vi "RT_Controller_Main.vi"() -> ()   [LabVIEW 2020]
uses:
  Components_global/DynamicSignalAnalyzer/TypeDefs/DSA_TF_Enum.ctl
  <vilib>/NI/STM/SubVIs/MetaDataElement.ctl
  <vilib>/NI/STM/TCP/TCP Write Options.ctl
  TypeDefs/STMLoopState_enum.ctl
  <vilib>/Platform/TimedLoop/XDataNode/timing_clust.ctl
  <vilib>/Platform/TimedLoop/XDataNode/nitl_modes.ctl
  <vilib>/Platform/TimedLoop/XDataNode/wakeup.ctl
  Components_global/PlannedMotionSequence/TypeDefs/PlannedMotionSequence.ctl
  Components_global/PlannedMotionSequence/TypeDefs/PlannedMotionSequence_Step.ctl
  Components_global/PlannedMotionSequence/TypeDefs/StepParams.ctl
  Components_global/PlannedMotionSequence/TypeDefs/CtrlEff Params.ctl
  Components_global/PlannedMotionSequence/TypeDefs/PosCtrl Params.ctl
  Components_global/PlannedMotionSequence/TypeDefs/HoldStateParams.ctl
  PC/Controller/TypeDefs/ControllerGains_UI.ctl
  PC/Controller/TypeDefs/ControllerGains_IndAxis.ctl
  Components_global/DynamicSignalAnalyzer/TypeDefs/DSAconfigCluster.ctl
  Components_global/DynamicSignalAnalyzer/TypeDefs/ExcitationSpecs.ctl
  Components_global/DynamicSignalAnalyzer/TypeDefs/CycleSpecs.ctl
  Components_global/DynamicSignalAnalyzer/TypeDefs/DSA_TF_params.ctl
  FPGA/Components/FPGA TypeDefs/SelectDirection_Enum.ctl
  <vilib>/NI/STM/TCP/TCP Read Options.ctl
  TypeDefs/FuncGenParams.ctl
  TypeDefs/SetRefLocEnum.ctl
  FPGA/Components/FPGA TypeDefs/SelectExcitation_Enum.ctl
  Components_global/Queues/InterProcessQueueCtl.ctl
  PC/Controller/TypeDefs/PosZeroOffsets.ctl
  <vilib>/Utility/error.llb/DialogType.ctl
  <vilib>/NI/STM/TCP/Write Meta Data (TCP Ref).vi
  <vilib>/NI/STM/TCP/Get Connection Reference (TCP).vi
  <vilib>/Analysis/2dsp.llb/Unwrap Phase.vi
  <vilib>/NI/STM/TCP/Write Meta Data (TCP Clst).vi
  <vilib>/FPGAPlugInAG/cRIO-9049/niLvFpga_Open_cRIO-9049.vi
  <vilib>/rvi/interface/common/dynamic/niFpgaDynamicAddResources.vi
  <vilib>/Utility/error.llb/Error Cluster From Error Code.vi
  <vilib>/rvi/errors/niLvFpgaAdjustHostInterfaceError.vi
  <vilib>/NI/STM/TCP/Write Message (TCP).vi
  Components_global/DynamicSignalAnalyzer/Private/Cycle_Calculator.vi
  Components_global/DynamicSignalAnalyzer/Private/Take_Data.vi
  Components_global/DynamicSignalAnalyzer/Private/System_Identify.vi
  Components_global/DynamicSignalAnalyzer/Private/Excitation_Gen.vi
  <vilib>/NI/STM/TCP/Read Message (TCP).vi
  <vilib>/FPGAPlugInAG/Dynamic/niLvFpga_Close_Dynamic.vi
  <vilib>/rvi/interface/nirviOpenFPGA/nirviOpenFPGA.xnode
  FPGA Bitfiles/levitationcode_FPGATarget_FPGAmainCtrlv3_XF-7iMJ+Fro.lvbitx
  <vilib>/Platform/TimedLoop/XDataNode/XDataNode.xnode
  <vilib>/rvi/interface/nirviReadWriteControl/nirviReadWriteControl.xnode
  <vilib>/rvi/interface/nirviCloseFPGA/nirviCloseFPGA.xnode
  <vilib>/NI/STM/NI STM.lvlib
  NiFpgaLv.dll
  Components_global/Timing/Timing.lvlib
  <vilib>/Platform/TimedLoop/XDataNode/XDNodeRunTimeDep.lvlib
  Components_global/Queues/Queues.lvlib
  Components_global/DynamicSignalAnalyzer/DynamicSignalAnalyzer.lvlib
  Components/FPGA control IO/FPGAcontrolIO.lvlib
  Components_global/PlannedMotionSequence/PlannedMotionSequence.lvlib
  <vilib>/rvi/interface/Simulation/niFpgaSimulationCallBeginRW.vi
panel:
  out "PlaMoS Iter. Dur. [us]":i64
  out "PlaMoSloop\nFinishedLate Counter":dbl
  out "DSA TF meas":T1
  out "Ts [s]":dbl caption="FPGA Ctrl Loop \nTime (Ts) [s]"
  out "DSAloop\nFinishedLate Counter":dbl
  out "DSAloop Iter. Dur. [us]":i64
  out "ReadLoop FinishedLate Counter":dbl
  out "ReadLoop Iteration \nDuration (us)":i64
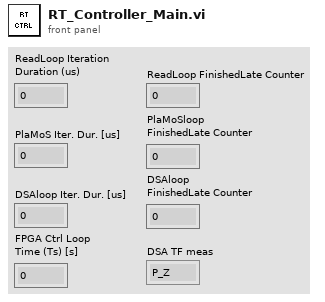
[diagram p1: front panel]
types:
  T1 = typedef "DynamicSignalAnalyzer.lvlib/DSA_TF_Enum.ctl" = enum16{"P_Z", "P_ThX", "P_ThY", "P_Bow", "P_B-d", "C_Z", "C_ThX", "C_ThY", "C_Bow", "C_B-d", "RR_Z", "RR_ThX", "RR_ThY", "RR_Bow", "RR_B-d", "*_custom"}
  T2 = typedef "STMLoopState_enum.ctl" = enum16{"Initialize", "Warm-up", "Run", "ShutDown"}
  T3 = typedef "NI STM.lvlib/TCP Write Options.ctl" = cluster{"ignore timeout error":bool, "timeout ms (1000)":i32}
  T4 = typedef "NI STM.lvlib/MetaDataElement.ctl" = string
  T5 = typedef "NI STM.lvlib/TCP Connection Info.ctl" = cluster{"connection ID":refnum<k5>, "meta data":T4[]}
  T6 = typedef "Queues.lvlib/Queue Refs.ctl" = cluster{"InterProcessQueue":refnum<queue>}
  T7 = typedef "XDNodeRunTimeDep.lvlib/timing_clust.ctl" = cluster{"Expected End [f-1]":u64, "Actual End [f-1]":u64, "Finished Late? [f-1]":bool, "Expected End [i-1]":u64, "Actual End [i-1]":u64, "Finished Late? [i-1]":bool, "Expected Start [i]":u64, "Actual Start [i]":u64, "Expected Start [f]":u64, "Actual Start [f]":u64, "Source Name":string, "Structure Name":string, "Period":i64, "Deadline":i64, "Offset":i64, "Start":i64, "Priority":i32, "Timeout":i32, "Mode":T8, "Wakeup Reason":T9, "Error":errorcluster, "Source Type":string, "Secondary Source Type":string, "Global End Time":u64, "Global Start Time":u64, "Frame Duration":u64, "Iteration Duration":u64, "Assigned CPU":i32, "I/O Scan Engine Mode":u32}
  T8 = typedef "XDNodeRunTimeDep.lvlib/nitl_modes.ctl" = enum32{"No Change", "Process missed periods, maintain original phase", "Discard missed periods, maintain original phase", "Process missed periods, ignore original phase", "Discard missed periods, ignore original phase"}
  T9 = typedef "XDNodeRunTimeDep.lvlib/wakeup.ctl" = enum32{"Normal", "Aborted", "Asynchronous wakeup", "Timing source error", "Timed loop error", "Timeout"}
  T10 = typedef "PlannedMotionSequence.lvlib/PlannedMotionSequence.ctl" = T11[]
  T11 = typedef "PlannedMotionSequence.lvlib/PlannedMotionSequence_Step.ctl" = cluster{"_Comment":string, "StepParams":T12, "Controller Gains":T16}
  T12 = typedef "PlannedMotionSequence.lvlib/StepParams.ctl" = cluster{"Ctrl State":enum16{"PosCtrl", "CtrlEff", "HoldState"}, "CtrlEff Params":T13, "PosCtrl Params":T14, "HoldState Params":T15}
  T13 = typedef "PlannedMotionSequence.lvlib/CtrlEff Params.ctl" = cluster{"Time [s]":dbl, "U_z":dbl}
  T14 = typedef "PlannedMotionSequence.lvlib/PosCtrl Params.ctl" = cluster{"Velocity [um/s]":dbl, "Starting Z-position [um]":dbl, "Ending Z-position [um]":dbl, "Bow Reference [um]":dbl}
  T15 = typedef "PlannedMotionSequence.lvlib/HoldStateParams.ctl" = cluster{"Time [s]":dbl}
  T16 = typedef "ControllerGains_UI.ctl" = cluster{"Z-direction":T17, "ThX-direction":T17, "ThY-direction":T17, "Bow-direction":T17, "Tor-direction":T17}
  T17 = typedef "ControllerGains_IndAxis.ctl" = cluster{"Kp":dbl, "Ki":dbl, "fLPF":dbl}
  T18 = cluster{"Period":i64, "State Index":i32, "index":i32}
  T19 = typedef "DynamicSignalAnalyzer.lvlib/DSAconfigCluster.ctl" = cluster{"DSA excitation specs":T20, "Cycle Specs":T21, "Meas. TF params":T22}
  T20 = typedef "DynamicSignalAnalyzer.lvlib/ExcitationSpecs.ctl" = cluster{"Initial Freq. [Hz]":dbl, "Final Freq. [Hz]":dbl, "# pts. in interval":i16, "Samping Time [us]":dbl, "Amplitude":dbl, "Offset [V]":dbl, "Freq Units (F: rad/s, T: Hz)":bool}
  T21 = typedef "DynamicSignalAnalyzer.lvlib/CycleSpecs.ctl" = cluster{"Cycles To \nSettle (M)":i16, "Cycles To \nCalculate (N)":i16}
  T22 = typedef "DynamicSignalAnalyzer.lvlib/DSA_TF_params.ctl" = cluster{"Direction":T23, "Tras. Func.":enum16{"P", "RR", "C", "*_custom"}}
  T23 = typedef "SelectDirection_Enum.ctl" = enum8{"Z", "ThX", "ThY", "Bow", "Tor"}
  T24 = typedef "NI STM.lvlib/TCP Read Options.ctl" = cluster{"ignore timeout error":bool, "timeout ms (1000)":i32}
  T25 = typedef "FuncGenParams.ctl" = cluster{"Reference Location":T26, "Direction":T23, "Excitation mode":T27, "Amplitude":dbl, "Frequency (periods/tick)":dbl, "PosRef_Offset":dbl[]}
  T26 = typedef "SetRefLocEnum.ctl" = enum16{"Pos Ref", "Ctrl Eff", "Elec Volt Dist"}
  T27 = typedef "SelectExcitation_Enum.ctl" = enum8{"DC", "Sine", "Square", "WhiteNoise"}
  T28 = typedef "Queues.lvlib/InterProcessQueueCtl.ctl" = cluster{"Command":string, "Data":variant}
  T29 = typedef "PosZeroOffsets.ctl" = cluster{"V_SE":dbl, "V_NE":dbl, "V_NW":dbl, "V_SW":dbl, "V_CI":dbl}
  T30 = cluster{"[0]":dbl, "[1]":dbl, "[2]":dbl, "[3]":dbl, "[4]":dbl}
  T31 = cluster{"[0]":dbl, "[1]":dbl, "[2]":dbl, "[3]":dbl, "[4]":dbl, "[5]":dbl}
  T32 = typedef "DialogType.ctl" = u16
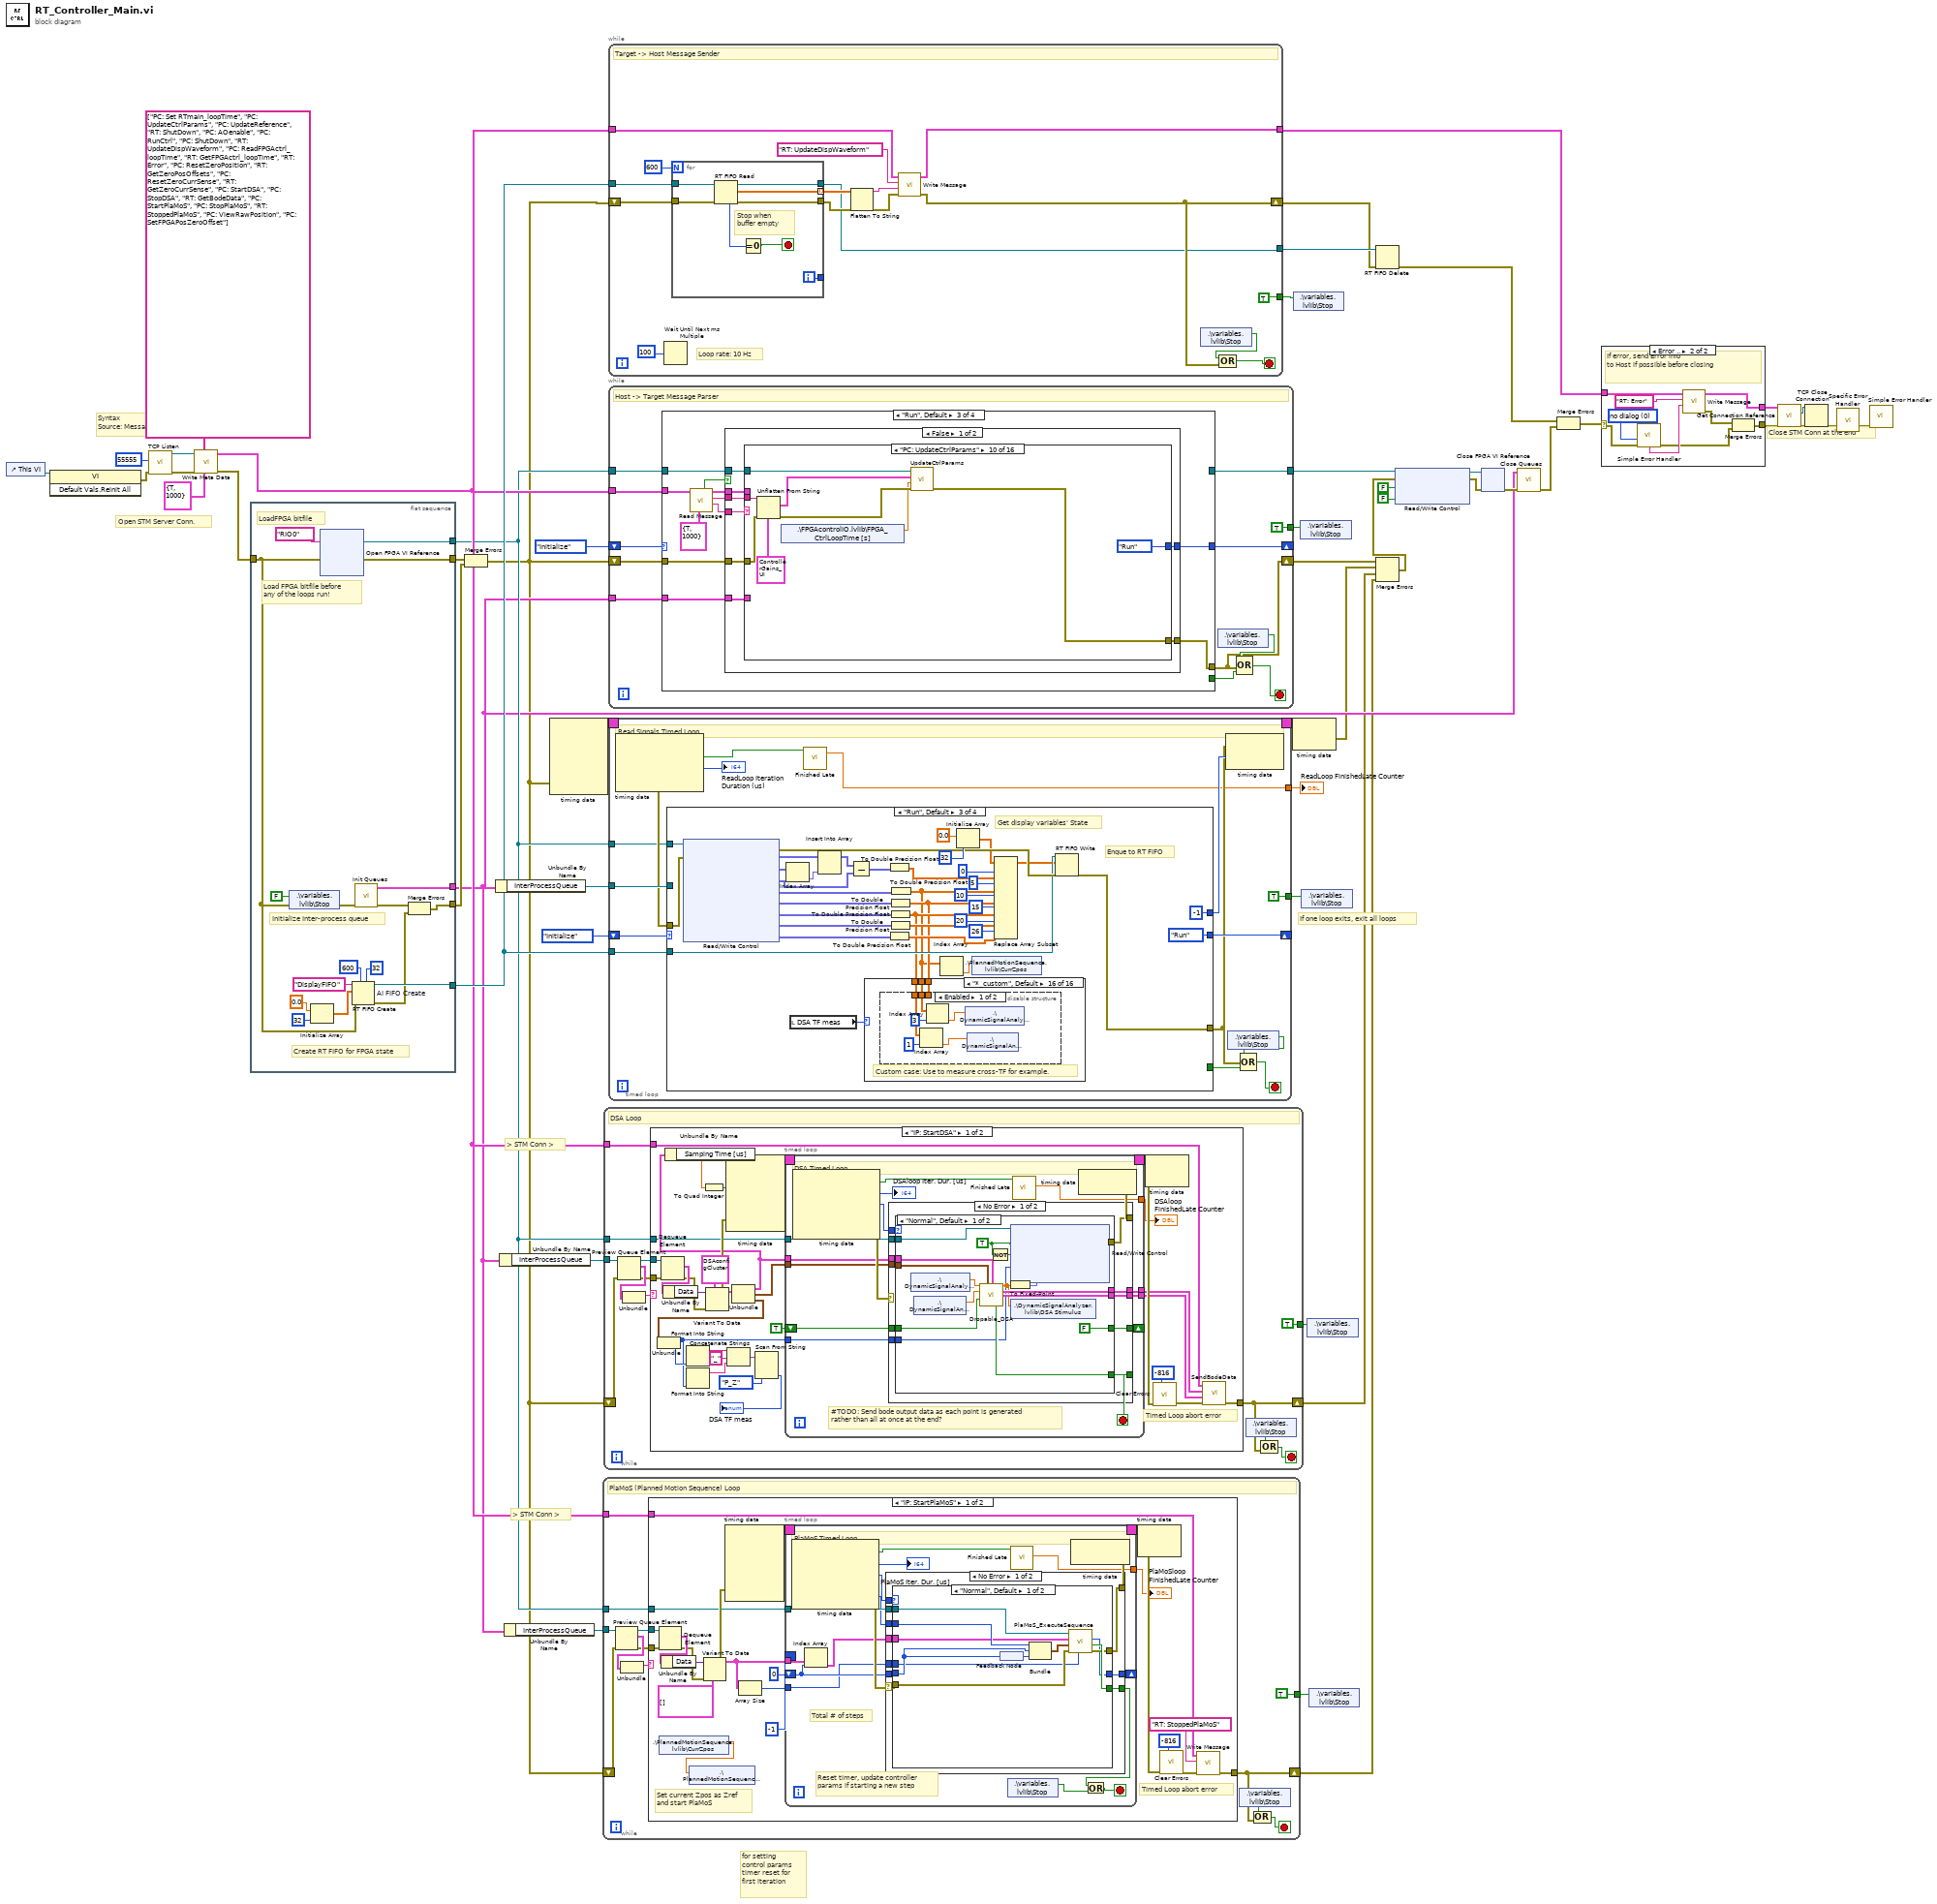
[diagram p0: block diagram]
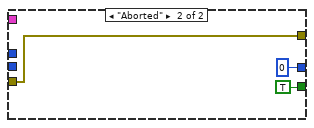
[diagram p2: hidden frame]
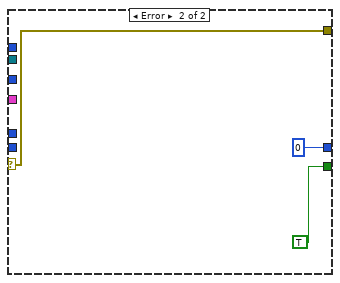
[diagram p3: hidden frame]
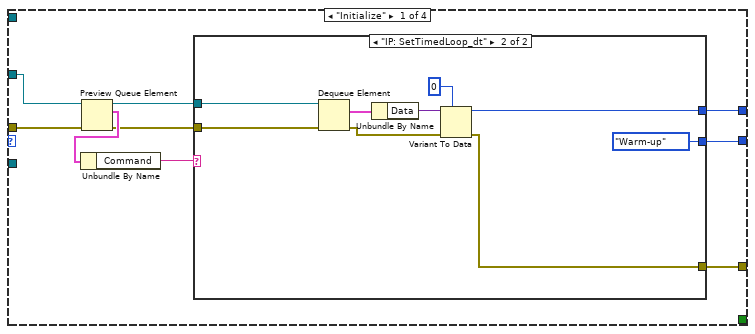
[diagram p5: hidden frame]
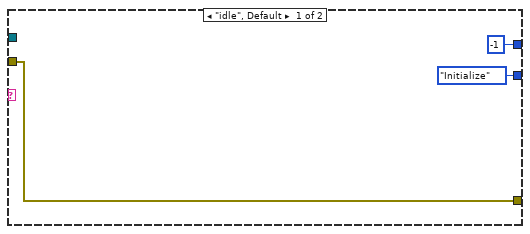
[diagram p6: hidden frame]
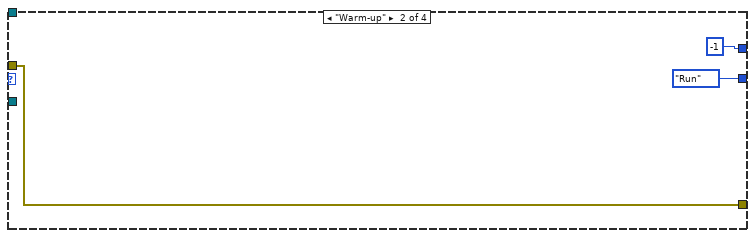
[diagram p7: hidden frame]
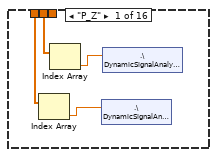
[diagram p8: hidden frame]
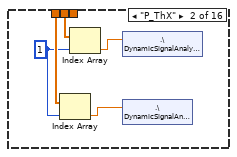
[diagram p9: hidden frame]
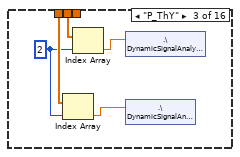
[diagram p10: hidden frame]
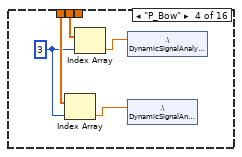
[diagram p11: hidden frame]
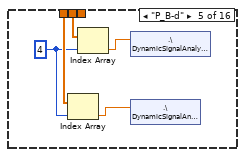
[diagram p12: hidden frame]
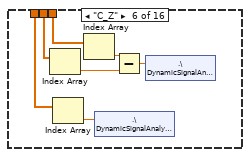
[diagram p13: hidden frame]
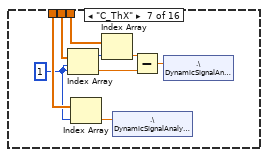
[diagram p14: hidden frame]
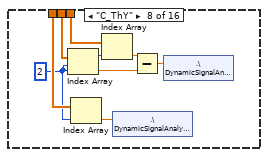
[diagram p15: hidden frame]
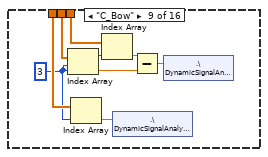
[diagram p16: hidden frame]
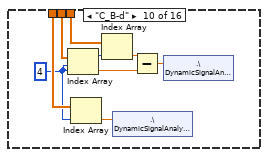
[diagram p17: hidden frame]
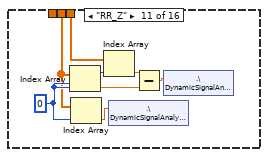
[diagram p18: hidden frame]
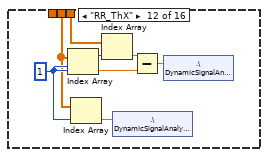
[diagram p19: hidden frame]
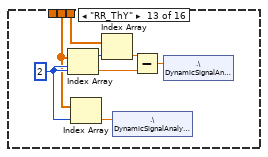
[diagram p20: hidden frame]
diagram:
  # "for setting control params\ntimer reset for\nfirst iteration"
  # "> STM Conn >"
  # "> STM Conn >"
  # "Close STM Conn at the end"
  # "Syntax\nSource: Message"
  # "Open STM Server Conn."
  # "If one loop exits, exit all loops"
  n1 = control-ref of="This VI"() -> (w13:refnum<vi>)
  n2 = invoke on="Invoke Node" class="VI" method="Default Vals.Reinit All"(reference=w13) -> (error out=w12:errorcluster)  [unwired: 2 in, 2 out]
  n3 = call <vilib>:"TCP Listen.vi"("error in (no error)"=w12, "port"=u16 55555) -> ("error out"=w50:errorcluster, "connection ID"=w49:refnum<k5>)  [unwired: 5 in, 3 out]
  n4 = call-poly <vilib>:"Write Meta Data.vi"("options"=T3 {"ignore timeout error"=TRUE, "timeout ms (1000)"=1000}, "meta data"=T4[] ["PC: Set RTmain_loopTime", "PC: UpdateCtrlParams", "PC: UpdateReference", "RT: ShutDown", "PC: AOenable", "PC: RunCtrl", "PC: ShutDown", "RT: UpdateDispWaveform", "PC: ReadFPGActrl_loopTime", "RT: GetFPGActrl_loopTime", "RT: Error", "PC: ResetZeroPosition", "RT: GetZeroPosOffsets", "PC: ResetZeroCurrSense", "RT: GetZeroCurrSense", "PC: StartDSA", "PC: StopDSA", "RT: GetBodeData", "PC: StartPlaMoS", "PC: StopPlaMoS", "RT: StoppedPlaMoS", "PC: ViewRawPosition", "PC: SetFPGAPosZeroOffset"], "error in"=w50, "connection ID"=w49) -> ("error out"=w45:errorcluster, "connection info out"=w9:T5)  [unwired: 1 in, 5 out]
  n5 = flat-sequence {
    tunnel: w45 -> [w53]
    tunnel: [w52] -> w8
    tunnel: [w68] -> w41
    tunnel: [w66] -> w6
    tunnel: [w56] -> w40
    tunnel: [w59] -> w36
    frame #0 {
      # "Create RT FIFO for FPGA state"
      # "LoadFPGA bitfile"
      # "Initialize Inter-process queue"
      # "Load FPGA bitfile before \nany of the loops run!"
      n6 = shared-variable ".\\variables.lvlib\\Stop"(FALSE ("Stop"), error in=w53) -> (error out=w58:errorcluster)
      n7 = Initialize Array(0.0 ("element"), 32 ("dimension size")) -> (w61:dbl[])
      n8 = xnode "Open FPGA VI Reference"("error in"=w53, "resource name"=tag "RIO0") -> ("FPGA VI Reference Out"=w52:refnum<k20>, "error out"=w68:errorcluster)
      n9 = RT FIFO Create "AI FIFO Create"(0:"DisplayFIFO" ("name (unnamed)"), 1:w61, 3:w53, 4:u32 600 ("size (10)"), 6:u32 32 ("elements in array (1)")) -> (8:w59:refnum<k33>, 11:w54:errorcluster)  [unwired: 3 in, 1 out]
      n10 = call "Init Queues.vi"("error in (no error)"=w58) -> ("error out"=w55:errorcluster, "Queue Refs"=w66:T6)  [unwired: 9 in]
      n11 = Merge Errors(w55, w54) -> (w56:errorcluster)
    }
  }
  n12 = Merge Errors(w41, w40) -> (w1:errorcluster)
  n13 = Unbundle By Name(w6) -> ("InterProcessQueue"=w39:refnum<queue>)
  n14 = Unbundle By Name(w6) -> ("InterProcessQueue"=w16:refnum<queue>)
  n15 = Unbundle By Name(w6) -> ("InterProcessQueue"=w11:refnum<queue>)
  n16 = node-c288(w1) -> (w44:T7)  [unwired: 4 in]
  n17 = while {
    tunnel: w11 -> [w80]
    tunnel: [TRUE ("Stop")] -> w10
    shift-right: [w71] -> w2
    shift-left: w1 -> [w73]
    tunnel: w9 -> [w70]
    tunnel: w8 -> [w69]
    stop <- w79 stop-if-true
    # "PlaMoS (Planned Motion Sequence) Loop"
    n18 = Preview Queue Element(queue=w80, error in (no error)=w73) -> (queue out=w74:refnum<queue>, element=w76:cluster{"Command":string, "Data":variant}, error out=w72:errorcluster)  [unwired: 1 in, 1 out]
    n19 = Unbundle(w76) -> ("Command"=w75:string)  [unwired: 1 out]
    n20 = case shown="\"IP: StartPlaMoS\"" w75 {
      tunnel: w74 -> [w100 _]
      tunnel: w72 -> [w99 w160]
      tunnel: [w91 w160] -> w71
      tunnel: w70 -> [w90 _]
      tunnel: w69 -> [w89 _]
      frame "IP: StartPlaMoS" {
        # "Set current Zpos as Zref \nand start PlaMoS"
        # "Timed Loop abort error"
        n21 = Dequeue Element(queue=w100, error in (no error)=w99) -> (element=w98:cluster{"Command":string, "Data":variant}, error out=w96:errorcluster)  [unwired: 1 in, 2 out]
        n22 = shared-variable ".\\PlannedMotionSequence.lvlib\\CurrZpos"() -> (w81:dbl)  [unwired: 1 in, 1 out]
        n23 = Unbundle By Name(w98) -> ("Data"=w97:variant)
        n24 = shared-variable ".\\PlannedMotionSequence.lvlib\\CurrZref"(w81) -> ()  [unwired: 1 in, 1 out]
        n25 = Variant To Data(error in=w96, type=T10 [] ("Planned Motion Sequence Steps"), Variant=w97) -> (data=w83:T10, error out=w95:errorcluster)
        n26 = node-c288(w95) -> (w102:T7)  [unwired: 4 in]
        n27 = Array Size(array=w83) -> (size(s)=w84:i32)
        n28 = timed-loop {
          timing: w102 -> [_]
          timing-out: [_] -> w101
          tunnel: w89 -> [w115]
          tunnel: [w113] -> w88
          tunnel: w83 -> [w108]
          shift-right: [w111] -> _
          shift-left: 0 ("State Index") -> [w109]
          tunnel: w84 -> [w107]
          border: -1 ("index") -> [_]
          stop <- w106 stop-if-true
          # "Reset timer, update controller params if starting a new step"
          # "Total # of steps"
          # "PlaMoS Timed Loop"
          n29 = node-c288() -> (w114:bool, →"PlaMoS Iter. Dur. [us]":i64, w118:T9, w117:errorcluster, w110:i64)  [unwired: 1 in]
          n30 = Index Array(array=w108, index=w109) -> (element=w103:T11)
          n31 = case shown="No Error" w117 {
            selector: w117 -> [w125 w145]
            tunnel: w118 -> [w128 _]
            tunnel: [w127 TRUE] -> w105
            tunnel: [w121 w145] -> w116
            tunnel: w115 -> [w126 _]
            tunnel: w109 -> [w124 _]
            tunnel: [w123 0 ("Next State Index")] -> w111
            tunnel: w110 -> [w122 _]
            tunnel: w107 -> [w120 _]
            tunnel: w103 -> [w119 _]
            frame No Error {
              n32 = case shown="\"Normal\", Default" w128 {
                tunnel: [w138 TRUE] -> w127
                tunnel: w126 -> [w134 _]
                tunnel: w125 -> [w139 w140]
                tunnel: w124 -> [w135 _]
                tunnel: [w131 0 ("Next State Index")] -> w123
                tunnel: w122 -> [w137 _]
                tunnel: [w133 w140] -> w121
                tunnel: w120 -> [w132 _]
                tunnel: w119 -> [w129 _]
                frame "Normal", Default {
                  n33 = feedback-in #1(w135) -> ()
                  n34 = feedback #1() -> (w130:i32)
                  n35 = Bundle("Period"=w137, "State Index"=w135, "index"=w130) -> (w136:T18)  [unwired: 1 in]
                  n36 = call "PlaMoS_ExecuteSequence.vi"("Total # of seq steps"=w132, "error in (no error)"=w139, "Curr Iter Params"=w136, "PlannedMotionSequence Step"=w129, "FPGA VI Reference In"=w134) -> ("error out"=w133:errorcluster, "PlaMoS completed?"=w138:bool, "Next State Index"=w131:i32)  [unwired: 3 in, 1 out]
                }
                frame "Aborted" {
                }
              }
            }
            frame Error {
            }
          }
          n37 = shared-variable ".\\variables.lvlib\\Stop"() -> (w104:bool)  [unwired: 1 in, 1 out]
          n38 = call "Finished Late.vi"("Finished \nLate?"=w114) -> ("# Finished\nLate counter"=w113:dbl)  [unwired: 8 in, 2 out]
          n39 = node-c288(w116) -> ()  [unwired: 1 out]
          n40 = Or(x=w105, y=w104) -> (x .or. y?=w106:bool)
        }
        "PlaMoSloop\nFinishedLate Counter" <- w88
        n41 = node-c288(w101) -> (w93:errorcluster)
        n42 = call <vilib>:"Clear Errors.vi"("error in (no error)"=w93, "specific error code to clear (0: all)"=-816) -> ("error out"=w92:errorcluster)  [unwired: 4 in, 1 out]
        n43 = call-poly <vilib>:"Write Message.vi"("error in"=w92, "name"="RT: StoppedPlaMoS", "connection info in"=w90) -> ("error out"=w91:errorcluster)  [unwired: 7 in, 1 out]
      }
      frame "idle", Default {
      }
    }
    n44 = shared-variable ".\\variables.lvlib\\Stop"() -> (w78:bool)  [unwired: 1 in, 1 out]
    n45 = Compound Arithmetic op=OR(w78, w71) -> (w79:bool)
  }
  n46 = while {
    tunnel: w16 -> [w172]
    tunnel: [TRUE ("Stop")] -> w15
    shift-right: [w163] -> w3
    shift-left: w1 -> [w165]
    tunnel: w9 -> [w162]
    tunnel: w8 -> [w161]
    stop <- w171 stop-if-true
    # "DSA Loop"
    n47 = Preview Queue Element(queue=w172, error in (no error)=w165) -> (queue out=w166:refnum<queue>, element=w168:cluster{"Command":string, "Data":variant}, error out=w164:errorcluster)  [unwired: 1 in, 1 out]
    n48 = Unbundle(w168) -> ("Command"=w167:string)  [unwired: 1 out]
    n49 = case shown="\"IP: StartDSA\"" w167 {
      tunnel: w166 -> [w203 _]
      tunnel: w164 -> [w202 w265]
      tunnel: [w187 w265] -> w163
      tunnel: w162 -> [w184 _]
      tunnel: w161 -> [w183 _]
      frame "IP: StartDSA" {
        # "Timed Loop abort error"
        n50 = Dequeue Element(queue=w203, error in (no error)=w202) -> (element=w201:cluster{"Command":string, "Data":variant}, error out=w198:errorcluster)  [unwired: 1 in, 2 out]
        n51 = Unbundle By Name(w201) -> ("Data"=w200:variant)
        n52 = Variant To Data(error in=w198, type=T19 {"DSA excitation specs"={"Initial Freq. [Hz]"=1.0, "Final Freq. [Hz]"=100.0, "# pts. in interval"=20, "Samping Time [us]"=0.0, "Amplitude"=0.0003, "Offset [V]"=0.0, "Freq Units (F: rad/s, T: Hz)"=TRUE}, "Cycle Specs"={"Cycles To \nSettle (M)"=1, "Cycles To \nCalculate (N)"=2}, "Meas. TF params"={"Direction"=enum."Z", "Tras. Func."=enum."P"}} ("DSA Config Cluster"), Variant=w200) -> (data=w195:T19, error out=w197:errorcluster)
        n53 = Unbundle(w195) -> ("DSA excitation specs"=w192:T20, "Cycle Specs"=w191:T21, "Meas. TF params"=w181:T22)
        n54 = Unbundle(w181) -> ("Direction"=w173:T23, "Tras. Func."=w180:enum16{"P", "RR", "C", "*_custom"})
        n55 = Unbundle By Name(w192) -> ("Samping Time [us]"=w189:dbl)
        n56 = Format Into String(w180) -> (resulting string=w179:string)  [unwired: 3 in, 1 out]
        n57 = Format Into String(w173) -> (resulting string=w177:string)  [unwired: 3 in, 1 out]
        n58 = To Quad Integer(1:w189) -> (0:w190:i64)
        n59 = node-c288(w190, w197) -> (w205:T7)  [unwired: 3 in]
        n60 = Concatenate Strings(w179, "_" ("string"), w177) -> (w176:string)
        n61 = Scan From String(input string=w176, default 1=DSA_TF_Enum."P_Z") -> (output 1=→"DSA TF meas":T1)  [unwired: 3 in, 3 out]
        n62 = timed-loop {
          timing: w205 -> [_]
          timing-out: [_] -> w204
          shift-right: [w215] -> _
          shift-left: TRUE ("START") -> [w216]
          tunnel: w192 -> [w214]
          tunnel: w191 -> [w213]
          tunnel: [w212] -> w186
          tunnel: [w211] -> w185
          tunnel: w183 -> [w209]
          tunnel: [w207] -> w182
          tunnel: w173 -> [w206]
          stop <- w219 stop-if-true
          # "#TODO: Send bode output data as each point is generated \nrather than all at once at the end?"
          # "DSA Timed Loop"
          n63 = node-c288() -> (w208:bool, →"DSAloop Iter. Dur. [us]":i64, w220:T9, w218:errorcluster)  [unwired: 1 in, 1 out]
          n64 = case shown="No Error" w218 {
            selector: w218 -> [_ w250]
            tunnel: w220 -> [w231 _]
            tunnel: [w230 TRUE] -> w219
            tunnel: [w222 w250] -> w217
            tunnel: w216 -> [w229 _]
            tunnel: [w228 _] -> w215
            tunnel: w214 -> [w227 _]
            tunnel: w213 -> [w226 _]
            tunnel: [w225 _] -> w212
            tunnel: [w224 _] -> w211
            tunnel: w209 -> [w223 _]
            tunnel: w206 -> [w221 _]
            frame No Error {
              n65 = case shown="\"Normal\", Default" w231 {
                tunnel: [w244 TRUE] -> w230
                tunnel: w229 -> [w243 _]
                tunnel: [FALSE ("START") _] -> w228
                tunnel: w227 -> [w242 _]
                tunnel: w226 -> [w241 _]
                tunnel: [w240 _] -> w225
                tunnel: [w239 _] -> w224
                tunnel: w223 -> [w238 _]
                tunnel: [w237 _] -> w222
                tunnel: w221 -> [w232 _]
                frame "Normal", Default {
                  w234 = TRUE ("Enable  Ctrl Eff dist?")
                  n66 = shared-variable ".\\DynamicSignalAnalyzer.lvlib\\TF Out"() -> (w247:dbl)  [unwired: 1 in, 1 out]
                  n67 = shared-variable ".\\DynamicSignalAnalyzer.lvlib\\TF In"() -> (w246:dbl)  [unwired: 1 in, 1 out]
                  n68 = call "Dropable_DSA.vi"("TF Out (CH B)"=w247, "Cycle Specs"=w241, "Excitation Specs"=w242, "TF In (CH A)"=w246, "START"=w243) -> ("Disturbance"=w236:dbl, "Bode Magnitude"=w240:cluster{dbl[], dbl[]}, "Bode Phase"=w239:cluster{dbl[], dbl[]}, "Stopped"=w244:bool)  [unwired: 5 in, 2 out]
                  n69 = Not(x=w234) -> (.not. x?=w235:bool)
                  n70 = To Fixed-Point(number=w236) -> (fixed-point=w233:fxp<+/-,25,5>)  [unwired: 1 in]
                  n71 = xnode "Read/Write Control"("FPGA VI Reference In"=w238, "Enable  Pos. Ref. Gen?"=w234, "Enable  Ctrl Eff dist?"=w235, "Select Ref. direction"=w232, "PR Amplitude [V]"=w233) -> ("error out"=w237:errorcluster)  [unwired: 1 in, 1 out]
                  n72 = shared-variable ".\\DynamicSignalAnalyzer.lvlib\\DSA Stimulus"(w236) -> ()  [unwired: 1 in, 1 out]
                }
                frame "Aborted" {
                }
              }
            }
            frame Error {
            }
          }
          n73 = call "Finished Late.vi"("Finished \nLate?"=w208) -> ("# Finished\nLate counter"=w207:dbl)  [unwired: 8 in, 2 out]
          n74 = node-c288(w217) -> ()  [unwired: 1 out]
        }
        "DSAloop\nFinishedLate Counter" <- w182
        n75 = node-c288(w204) -> (w193:errorcluster)
        n76 = call <vilib>:"Clear Errors.vi"("error in (no error)"=w193, "specific error code to clear (0: all)"=-816) -> ("error out"=w188:errorcluster)  [unwired: 4 in, 1 out]
        n77 = call "SendBodeData.vi"("error in (no error)"=w188, "Phase Array"=w185, "Magnitude Array"=w186, "connection info in"=w184) -> ("error out"=w187:errorcluster)  [unwired: 6 in, 1 out]
      }
      frame "idle", Default {
      }
    }
    n78 = shared-variable ".\\variables.lvlib\\Stop"() -> (w170:bool)  [unwired: 1 in, 1 out]
    n79 = Compound Arithmetic op=OR(w170, w163) -> (w171:bool)
  }
  n80 = timed-loop {
    timing: w44 -> [_]
    timing-out: [_] -> w43
    shift-right: [w279] -> _
    shift-left: STMLoopState_enum."Initialize" ("RTmainLoopState") -> [w280]
    tunnel: w39 -> [w276]
    tunnel: [TRUE ("Stop")] -> w38
    tunnel: w36 -> [w268]
    tunnel: w8 -> [w267]
    tunnel: [w266] -> w18
    stop <- w273 stop-if-true
    # "Read Signals Timed Loop"
    n81 = node-c288() -> (w274:errorcluster, w278:bool, →"ReadLoop Iteration \nDuration (us)":i64)  [unwired: 1 in, 1 out]
    n82 = case shown="\"Run\", Default" w280 {
      tunnel: [w286 STMLoopState_enum."Run" ("RTmainLoopState") STMLoopState_enum."Run" ("RTmainLoopState") STMLoopState_enum."ShutDown" ("RTmainLoopState")] -> w279
      tunnel: [_ _ _ TRUE] -> w272
      tunnel: w276 -> [w285 _ _ _]
      tunnel: [w284 i64 -1 ("Period") i64 -1 ("Period") i64 1000 ("Period")] -> w275
      tunnel: w274 -> [w283 w302 w337 w456]
      tunnel: [w281 w302 w330 w456] -> w271
      tunnel: w268 -> [_ _ w329 _]
      tunnel: w267 -> [_ _ w338 _]
      frame "Initialize" {
        n83 = Preview Queue Element(queue=w285, error in (no error)=w283) -> (queue out=w289:refnum<queue>, element=w288:cluster{"Command":string, "Data":variant}, error out=w282:errorcluster)  [unwired: 1 in, 1 out]
        n84 = Unbundle By Name(w288) -> ("Command"=w287:string)
        n85 = case shown="\"IP: SetTimedLoop_dt\"" w287 {
          tunnel: w289 -> [_ w300]
          tunnel: [STMLoopState_enum."Initialize" ("RTmainLoopState") STMLoopState_enum."Warm-up" ("RTmainLoopState")] -> w286
          tunnel: [i64 -1 w296] -> w284
          tunnel: w282 -> [w290 w295]
          tunnel: [w290 w293] -> w281
          frame "idle", Default {
          }
          frame "IP: SetTimedLoop_dt" {
            n86 = Dequeue Element(queue=w300, error in (no error)=w295) -> (element=w299:cluster{"Command":string, "Data":variant}, error out=w294:errorcluster)  [unwired: 1 in, 2 out]
            n87 = Unbundle By Name(w299) -> ("Data"=w298:variant)
            n88 = Variant To Data(error in=w294, type=i64 0, Variant=w298) -> (data=w296:i64, error out=w293:errorcluster)
          }
        }
      }
      frame "Warm-up" {
      }
      frame "Run", Default {
        # "Enque to RT FIFO"
        # "Get display variables' State"
        n89 = xnode "Read/Write Control"("FPGA VI Reference In"=w338, "error in"=w337) -> ("error out"=w331:errorcluster, "AI_HS"=w325:fxp<+/-,25,5>[], "AI_LS"=w327:fxp<+/-,25,5>[], "PosMeas_ZeroOffset"=w326:fxp<+/-,25,5>[], "Z,ThX,ThY,B,Bd Meas"=w310:fxp<+/-,25,5>[], "Total PosRef"=w336:fxp<+/-,25,5>[], "Total Ctrl Eff"=w335:fxp<+/-,25,5>[], "AO"=w334:fxp<+/-,20,5>[], "Current Sense"=w328:fxp<+/-,25,5>[])  [unwired: 1 out]
        n90 = Index Array(array=w327) -> (element=w324:fxp<+/-,25,5>)  [unwired: 1 in]
        n91 = local read "DSA TF meas"() -> (w307:T1)
        n92 = Insert Into Array(array=w325, new element=w324) -> (w323:fxp<+/-,25,5>[])  [unwired: 1 in]
        n93 = Subtract(x=w323, y=w326) -> (x-y=w322:fxp<+/-,26,6>[])
        n94 = To Double Precision Float(number=w322) -> (double precision float=w320:dbl[])
        n95 = To Double Precision Float(number=w328) -> (double precision float=w313:dbl[])
        n96 = To Double Precision Float(number=w336) -> (double precision float=w308:dbl[])
        n97 = To Double Precision Float(number=w335) -> (double precision float=w309:dbl[])
        n98 = To Double Precision Float(number=w334) -> (double precision float=w314:dbl[])
        n99 = To Double Precision Float(number=w310) -> (double precision float=w305:dbl[])
        n100 = case shown="\"*_custom\", Default" w307 {
          tunnel: w305 -> [w343 w348 w353 w358 w363 w371 w379 w387 w395 w403 w404 w411 w418 w425 w432 w441]
          tunnel: w309 -> [w341 w346 w351 w356 w361 w365 w373 w381 w389 w397 _ _ _ _ _ w440]
          tunnel: w308 -> [_ _ _ _ _ w367 w375 w383 w391 w399 w407 w414 w421 w428 w435 w439]
          frame "P_Z" {
            n101 = Index Array(array=w341) -> (element=w342:dbl)  [unwired: 1 in]
            n102 = Index Array(array=w343) -> (element=w344:dbl)  [unwired: 1 in]
            n103 = shared-variable ".\\DynamicSignalAnalyzer.lvlib\\TF In"(w342) -> ()  [unwired: 1 in, 1 out]
            n104 = shared-variable ".\\DynamicSignalAnalyzer.lvlib\\TF Out"(w344) -> ()  [unwired: 1 in, 1 out]
          }
          frame "P_ThX" {
            w345 = 1 ("index")
            n105 = Index Array(array=w346, index=w345) -> (element=w347:dbl)
            n106 = Index Array(array=w348, index=w345) -> (element=w349:dbl)
            n107 = shared-variable ".\\DynamicSignalAnalyzer.lvlib\\TF Out"(w349) -> ()  [unwired: 1 in, 1 out]
            n108 = shared-variable ".\\DynamicSignalAnalyzer.lvlib\\TF In"(w347) -> ()  [unwired: 1 in, 1 out]
          }
          frame "P_ThY" {
            w350 = 2 ("index")
            n109 = Index Array(array=w351, index=w350) -> (element=w352:dbl)
            n110 = Index Array(array=w353, index=w350) -> (element=w354:dbl)
            n111 = shared-variable ".\\DynamicSignalAnalyzer.lvlib\\TF Out"(w354) -> ()  [unwired: 1 in, 1 out]
            n112 = shared-variable ".\\DynamicSignalAnalyzer.lvlib\\TF In"(w352) -> ()  [unwired: 1 in, 1 out]
          }
          frame "P_Bow" {
            w355 = 3 ("index")
            n113 = Index Array(array=w356, index=w355) -> (element=w357:dbl)
            n114 = Index Array(array=w358, index=w355) -> (element=w359:dbl)
            n115 = shared-variable ".\\DynamicSignalAnalyzer.lvlib\\TF Out"(w359) -> ()  [unwired: 1 in, 1 out]
            n116 = shared-variable ".\\DynamicSignalAnalyzer.lvlib\\TF In"(w357) -> ()  [unwired: 1 in, 1 out]
          }
          frame "P_B-d" {
            w360 = 4 ("index")
            n117 = Index Array(array=w361, index=w360) -> (element=w362:dbl)
            n118 = Index Array(array=w363, index=w360) -> (element=w364:dbl)
            n119 = shared-variable ".\\DynamicSignalAnalyzer.lvlib\\TF Out"(w364) -> ()  [unwired: 1 in, 1 out]
            n120 = shared-variable ".\\DynamicSignalAnalyzer.lvlib\\TF In"(w362) -> ()  [unwired: 1 in, 1 out]
          }
          frame "C_Z" {
            n121 = Index Array(array=w371) -> (element=w366:dbl)  [unwired: 1 in]
            n122 = Index Array(array=w365) -> (element=w370:dbl)  [unwired: 1 in]
            n123 = Index Array(array=w367) -> (element=w368:dbl)  [unwired: 1 in]
            n124 = shared-variable ".\\DynamicSignalAnalyzer.lvlib\\TF Out"(w370) -> ()  [unwired: 1 in, 1 out]
            n125 = Subtract(x=w368, y=w366) -> (x-y=w369:dbl)
            n126 = shared-variable ".\\DynamicSignalAnalyzer.lvlib\\TF In"(w369) -> ()  [unwired: 1 in, 1 out]
          }
          frame "C_ThX" {
            w372 = 1 ("index")
            n127 = Index Array(array=w379, index=w372) -> (element=w374:dbl)
            n128 = Index Array(array=w373, index=w372) -> (element=w378:dbl)
            n129 = Index Array(array=w375, index=w372) -> (element=w376:dbl)
            n130 = shared-variable ".\\DynamicSignalAnalyzer.lvlib\\TF Out"(w378) -> ()  [unwired: 1 in, 1 out]
            n131 = Subtract(x=w376, y=w374) -> (x-y=w377:dbl)
            n132 = shared-variable ".\\DynamicSignalAnalyzer.lvlib\\TF In"(w377) -> ()  [unwired: 1 in, 1 out]
          }
          frame "C_ThY" {
            w380 = 2 ("index")
            n133 = Index Array(array=w387, index=w380) -> (element=w382:dbl)
            n134 = Index Array(array=w381, index=w380) -> (element=w386:dbl)
            n135 = Index Array(array=w383, index=w380) -> (element=w384:dbl)
            n136 = shared-variable ".\\DynamicSignalAnalyzer.lvlib\\TF Out"(w386) -> ()  [unwired: 1 in, 1 out]
            n137 = Subtract(x=w384, y=w382) -> (x-y=w385:dbl)
            n138 = shared-variable ".\\DynamicSignalAnalyzer.lvlib\\TF In"(w385) -> ()  [unwired: 1 in, 1 out]
          }
          frame "C_Bow" {
            w388 = 3 ("index")
            n139 = Index Array(array=w395, index=w388) -> (element=w390:dbl)
            n140 = Index Array(array=w389, index=w388) -> (element=w394:dbl)
            n141 = Index Array(array=w391, index=w388) -> (element=w392:dbl)
            n142 = shared-variable ".\\DynamicSignalAnalyzer.lvlib\\TF Out"(w394) -> ()  [unwired: 1 in, 1 out]
            n143 = Subtract(x=w392, y=w390) -> (x-y=w393:dbl)
            n144 = shared-variable ".\\DynamicSignalAnalyzer.lvlib\\TF In"(w393) -> ()  [unwired: 1 in, 1 out]
          }
          frame "C_B-d" {
            w396 = 4 ("index")
            n145 = Index Array(array=w403, index=w396) -> (element=w398:dbl)
            n146 = Index Array(array=w397, index=w396) -> (element=w402:dbl)
            n147 = Index Array(array=w399, index=w396) -> (element=w400:dbl)
            n148 = shared-variable ".\\DynamicSignalAnalyzer.lvlib\\TF Out"(w402) -> ()  [unwired: 1 in, 1 out]
            n149 = Subtract(x=w400, y=w398) -> (x-y=w401:dbl)
            n150 = shared-variable ".\\DynamicSignalAnalyzer.lvlib\\TF In"(w401) -> ()  [unwired: 1 in, 1 out]
          }
          frame "RR_Z" {
            w405 = 0 ("index")
            n151 = Index Array(array=w404, index=w405) -> (element=w406:dbl)
            n152 = Index Array(array=w404, index=w405) -> (element=w410:dbl)
            n153 = Index Array(array=w407, index=w405) -> (element=w408:dbl)
            n154 = shared-variable ".\\DynamicSignalAnalyzer.lvlib\\TF Out"(w410) -> ()  [unwired: 1 in, 1 out]
            n155 = Subtract(x=w408, y=w406) -> (x-y=w409:dbl)
            n156 = shared-variable ".\\DynamicSignalAnalyzer.lvlib\\TF In"(w409) -> ()  [unwired: 1 in, 1 out]
          }
          frame "RR_ThX" {
            w412 = 1 ("index")
            n157 = Index Array(array=w411, index=w412) -> (element=w413:dbl)
            n158 = Index Array(array=w411, index=w412) -> (element=w417:dbl)
            n159 = Index Array(array=w414, index=w412) -> (element=w415:dbl)
            n160 = shared-variable ".\\DynamicSignalAnalyzer.lvlib\\TF Out"(w417) -> ()  [unwired: 1 in, 1 out]
            n161 = Subtract(x=w415, y=w413) -> (x-y=w416:dbl)
            n162 = shared-variable ".\\DynamicSignalAnalyzer.lvlib\\TF In"(w416) -> ()  [unwired: 1 in, 1 out]
          }
          frame "RR_ThY" {
            w419 = 2 ("index")
            n163 = Index Array(array=w418, index=w419) -> (element=w420:dbl)
            n164 = Index Array(array=w418, index=w419) -> (element=w424:dbl)
            n165 = Index Array(array=w421, index=w419) -> (element=w422:dbl)
            n166 = shared-variable ".\\DynamicSignalAnalyzer.lvlib\\TF Out"(w424) -> ()  [unwired: 1 in, 1 out]
            n167 = Subtract(x=w422, y=w420) -> (x-y=w423:dbl)
            n168 = shared-variable ".\\DynamicSignalAnalyzer.lvlib\\TF In"(w423) -> ()  [unwired: 1 in, 1 out]
          }
          frame "RR_Bow" {
            w426 = 3 ("index")
            n169 = Index Array(array=w425, index=w426) -> (element=w427:dbl)
            n170 = Index Array(array=w425, index=w426) -> (element=w431:dbl)
            n171 = Index Array(array=w428, index=w426) -> (element=w429:dbl)
            n172 = shared-variable ".\\DynamicSignalAnalyzer.lvlib\\TF Out"(w431) -> ()  [unwired: 1 in, 1 out]
            n173 = Subtract(x=w429, y=w427) -> (x-y=w430:dbl)
            n174 = shared-variable ".\\DynamicSignalAnalyzer.lvlib\\TF In"(w430) -> ()  [unwired: 1 in, 1 out]
          }
          frame "RR_B-d" {
            w433 = 4 ("index")
            n175 = Index Array(array=w432, index=w433) -> (element=w434:dbl)
            n176 = Index Array(array=w432, index=w433) -> (element=w438:dbl)
            n177 = Index Array(array=w435, index=w433) -> (element=w436:dbl)
            n178 = shared-variable ".\\DynamicSignalAnalyzer.lvlib\\TF Out"(w438) -> ()  [unwired: 1 in, 1 out]
            n179 = Subtract(x=w436, y=w434) -> (x-y=w437:dbl)
            n180 = shared-variable ".\\DynamicSignalAnalyzer.lvlib\\TF In"(w437) -> ()  [unwired: 1 in, 1 out]
          }
          frame "*_custom", Default {
            # "Custom case: Use to measure cross-TF for example."
            n181 = disable-structure shown="Enabled" {
              disable-tunnel: w441 -> [w446 w450]
              disable-tunnel: w440 -> [w444 _]
              disable-tunnel: w439 -> [_ w449]
              frame Enabled {
                n182 = Index Array(array=w444, index=1) -> (element=w445:dbl)
                n183 = Index Array(array=w446, index=3) -> (element=w447:dbl)
                n184 = shared-variable ".\\DynamicSignalAnalyzer.lvlib\\TF Out"(w447) -> ()  [unwired: 1 in, 1 out]
                n185 = shared-variable ".\\DynamicSignalAnalyzer.lvlib\\TF In"(w445) -> ()  [unwired: 1 in, 1 out]
              }
              frame Disabled {
                w448 = 1 ("index")
                n186 = Index Array(array=w450, index=w448) -> (element=w452:dbl)
                n187 = Index Array(array=w450, index=4) -> (element=w455:dbl)
                n188 = Index Array(array=w449, index=w448) -> (element=w453:dbl)
                n189 = shared-variable ".\\DynamicSignalAnalyzer.lvlib\\TF Out"(w455) -> ()  [unwired: 1 in, 1 out]
                n190 = Subtract(x=w453, y=w452) -> (x-y=w454:dbl)
                n191 = shared-variable ".\\DynamicSignalAnalyzer.lvlib\\TF In"(w454) -> ()  [unwired: 1 in, 1 out]
              }
            }
          }
        }
        n192 = Index Array(array=w305) -> (element=w306:dbl)  [unwired: 1 in]
        n193 = Initialize Array(0.0 ("element"), 32 ("dimension size")) -> (w312:dbl[])
        n194 = shared-variable ".\\PlannedMotionSequence.lvlib\\CurrZpos"(w306) -> ()  [unwired: 1 in, 1 out]
        n195 = Replace Array Subset(array=w312, new element #1=w320, index #1=0 ("index"), new element #2=w305, index #2=5 ("index"), new element #3=w308, index #3=10 ("index"), new element #4=w309, index #4=15 ("index"), new element #5=w314, index #5=20 ("index"), new element #6=w313, index #6=26 ("index")) -> (w311:dbl[])
        n196 = RT FIFO Write(0:w329, 1:w311, 3:w331) -> (11:w330:errorcluster)  [unwired: 2 in, 3 out]
      }
      frame "ShutDown" {
      }
    }
    n197 = call "Finished Late.vi"("Finished \nLate?"=w278) -> ("# Finished\nLate counter"=w266:dbl)  [unwired: 8 in, 2 out]
    n198 = node-c288(w271, w275) -> ()  [unwired: 1 out]
    n199 = shared-variable ".\\variables.lvlib\\Stop"() -> (w269:bool)  [unwired: 1 in, 1 out]
    n200 = Compound Arithmetic op=OR(w269, w271, w272) -> (w273:bool)
  }
  "ReadLoop FinishedLate Counter" <- w18
  n201 = while {
    tunnel: w36 -> [w483]
    tunnel: w9 -> [w480]
    tunnel: [w471] -> w21
    tunnel: [w470] -> w35
    tunnel: [TRUE ("Stop")] -> w17
    shift-right: [w473] -> w29
    shift-left: w1 -> [w468]
    stop <- w472 stop-if-true
    # "Loop rate: 10 Hz"
    # "Target -> Host Message Sender"
    n202 = Wait Until Next ms Multiple(millisecond multiple=u32 100) -> ()  [unwired: 1 out]
    n203 = for {
      N: 600 -> [_]
      tunnel: w483 -> [w491]
      tunnel: [w488] -> w478 mode=indexing
      tunnel: w468 -> [w487]
      tunnel: [w486] -> w476
      tunnel: [w485] -> w470
      tunnel: [w484] -> _
      i -> [w484]
      stop <- w489 stop-if-true
      # "Stop when\nbuffer empty"
      n204 = RT FIFO Read(0:w491, 3:w487) -> (7:w490:u32, 8:w485:refnum<k33>, 9:w488:dbl[], 11:w486:errorcluster)  [unwired: 2 in, 1 out]
      n205 = Equal To 0?(x=w490) -> (x = 0?=w489:bool)
    }
    n206 = Flatten To String(anything=w478, error in (no error)=w476) -> (data string=w477:string, error out=w475:errorcluster)  [unwired: 2 in, 1 out]
    n207 = call-poly <vilib>:"Write Message.vi"("error in"=w475, "data"=w477, "name"="RT: UpdateDispWaveform", "connection info in"=w480) -> ("error out"=w473:errorcluster, "connection info out"=w471:T5)  [unwired: 6 in]
    n208 = shared-variable ".\\variables.lvlib\\Stop"() -> (w474:bool)  [unwired: 1 in, 1 out]
    n209 = Compound Arithmetic op=OR(w474, w473) -> (w472:bool)
  }
  n210 = while {
    shift-right: [w501] -> _
    shift-left: STMLoopState_enum."Initialize" ("RTmainLoopState") -> [w503]
    tunnel: w9 -> [w502]
    tunnel: w8 -> [w498]
    tunnel: w6 -> [w496]
    tunnel: [TRUE ("Stop")] -> w37
    tunnel: [w493] -> w24
    shift-right: [w492] -> w14
    shift-left: w1 -> [w497]
    stop <- w499 stop-if-true
    # "Host -> Target Message Parser"
    n211 = case shown="\"Run\", Default" w503 {
      tunnel: w502 -> [_ _ w520 w756]
      tunnel: [STMLoopState_enum."Run" ("RTmainLoopState") STMLoopState_enum."Run" ("RTmainLoopState") w514 STMLoopState_enum."ShutDown" ("RTmainLoopState")] -> w501
      tunnel: [_ _ _ TRUE] -> w500
      tunnel: [w505 _ w518 w753] -> w492
      tunnel: w498 -> [w509 _ w519 w757]
      tunnel: w497 -> [w508 _ w516 w755]
      tunnel: w496 -> [_ _ w512 _]
      tunnel: [_ _ _ w757] -> w493
      frame "Initialize" {
        n212 = xnode "Read/Write Control"("FPGA VI Reference In"=w509, "error in"=w508) -> ("error out"=w505:errorcluster, "Ctrl Loop time [ticks]"=w507:u32)  [unwired: 1 out]
        n213 = Multiply(x=w507, y=2.5e-08) -> (x*y=w504:dbl)
        "Ts [s]" <- w504
        n214 = shared-variable ".\\FPGAcontrolIO.lvlib\\FPGA_CtrlLoopTime [s]"(w504) -> ()  [unwired: 1 in, 1 out]
      }
      frame "Warm-up" {
      }
      frame "Run", Default {
        n215 = call-poly <vilib>:"Read Message.vi"("options"=T24 {"ignore timeout error"=TRUE, "timeout ms (1000)"=1000}, "connection info in"=w520) -> ("name"=w522:T4, "data string"=w521:string, "connection info out"=w513:T5, "timed out?"=w517:bool)  [unwired: 3 in, 3 out]
        n216 = case shown="False" w517 {
          tunnel: w522 -> [w530 _]
          tunnel: w521 -> [w529 _]
          tunnel: w519 -> [w528 _]
          tunnel: [w527 w747] -> w518
          tunnel: w516 -> [w526 w747]
          tunnel: [w525 STMLoopState_enum."Run" ("RTmainLoopState")] -> w514
          tunnel: w513 -> [w524 _]
          tunnel: w512 -> [w523 _]
          frame False {
            n217 = case shown="\"PC: UpdateCtrlParams\"" w530 {
              tunnel: w529 -> [w537 _ _ w557 _ _ _ w615 _ w678 w683 w703 w718 _ w733 _]
              tunnel: w528 -> [w533 _ w553 w558 w579 w591 w606 w611 w661 w670 _ w698 w716 _ _ _]
              tunnel: [w534 w540 w542 w555 w566 w584 w597 w608 w654 w672 w679 w692 w715 w723 w728 w742] -> w527
              tunnel: w526 -> [w532 w540 w552 w556 _ w581 _ w609 w658 w677 w680 w700 w717 w726 w730 w745]
              tunnel: [STMLoopState_enum."Run" ("RTmainLoopState") STMLoopState_enum."Run" ("RTmainLoopState") STMLoopState_enum."Run" ("RTmainLoopState") STMLoopState_enum."Run" ("RTmainLoopState") STMLoopState_enum."Run" ("RTmainLoopState") STMLoopState_enum."Run" ("RTmainLoopState") STMLoopState_enum."Run" ("RTmainLoopState") STMLoopState_enum."Run" ("RTmainLoopState") STMLoopState_enum."ShutDown" ("RTmainLoopState") STMLoopState_enum."Run" ("RTmainLoopState") STMLoopState_enum."Run" ("RTmainLoopState") STMLoopState_enum."Run" ("RTmainLoopState") STMLoopState_enum."Run" ("RTmainLoopState") STMLoopState_enum."Run" ("RTmainLoopState") STMLoopState_enum."Run" ("RTmainLoopState") STMLoopState_enum."Run" ("RTmainLoopState")] -> w525
              tunnel: w524 -> [_ _ w545 _ w568 w586 w599 _ _ _ _ _ _ _ _ _]
              tunnel: w523 -> [_ _ _ _ _ _ _ _ w656 _ w682 w702 _ _ w732 _]
              frame "PC: AOenable" {
                n218 = Unflatten From String(type=FALSE, binary string=w537, error in (no error)=w532) -> (value=w536:bool, error out=w535:errorcluster)  [unwired: 2 in, 1 out]
                n219 = xnode "Read/Write Control"("FPGA VI Reference In"=w533, "error in"=w535, "AO enable?"=w536) -> ("error out"=w534:errorcluster)  [unwired: 1 out]
              }
              frame "idle", Default {
              }
              frame "PC: ReadFPGActrl_loopTime" {
                # "SendCtrlLoop time in us"
                n220 = xnode "Read/Write Control"("FPGA VI Reference In"=w553, "error in"=w552) -> ("error out"=w547:errorcluster, "Ctrl Loop time [ticks]"=w549:u32)  [unwired: 1 out]
                n221 = To Double Precision Float(number=w549) -> (double precision float=w550:dbl)
                n222 = Multiply(x=w550, y=0.025) -> (x*y=w548:dbl)
                n223 = Flatten To String(anything=w548, error in (no error)=w547) -> (data string=w546:string, error out=w543:errorcluster)  [unwired: 2 in, 1 out]
                n224 = call-poly <vilib>:"Write Message.vi"("error in"=w543, "data"=w546, "name"="RT: GetFPGActrl_loopTime", "connection info in"=w545) -> ("error out"=w542:errorcluster)  [unwired: 6 in, 1 out]
              }
              frame "PC: RunCtrl" {
                n225 = Unflatten From String(type=FALSE, binary string=w557, error in (no error)=w556) -> (value=w560:bool, error out=w559:errorcluster)  [unwired: 2 in, 1 out]
                n226 = xnode "Read/Write Control"("FPGA VI Reference In"=w558, "error in"=w559, "Run Controller?"=w560) -> ("error out"=w555:errorcluster)  [unwired: 1 out]
              }
              frame "PC: ResetZeroPosition" {
                n227 = xnode "Read/Write Control"("FPGA VI Reference In"=w579) -> ("FPGA VI Reference Out"=w576:refnum<k20>, "error out"=w577:errorcluster, "AI_HS"=w573:fxp<+/-,25,5>[], "AI_LS"=w575:fxp<+/-,25,5>[])  [unwired: 1 in]
                n228 = Index Array(array=w575) -> (element=w572:fxp<+/-,25,5>)  [unwired: 1 in]
                n229 = Replace Array Subset(array=fxp<+/-,25,5>[] [0.0, 0.0, 0.0, 0.0, 0.0] ("PosMeas_ZeroOffset"), new element #1=w573, new element #2=w572, index #2=4 ("index")) -> (w565:fxp<+/-,25,5>[])  [unwired: 1 in]
                n230 = To Double Precision Float(number=w565) -> (double precision float=w564:dbl[])
                n231 = xnode "Read/Write Control"("FPGA VI Reference In"=w576, "error in"=w577, "PosMeas_ZeroOffset"=w565) -> ("error out"=w567:errorcluster)  [unwired: 1 out]
                n232 = Array To Cluster(array=w564) -> (cluster=w563:T30)
                n233 = Flatten To String(anything=w563, error in (no error)=w567) -> (data string=w571:string, error out=w569:errorcluster)  [unwired: 2 in, 1 out]
                n234 = call-poly <vilib>:"Write Message.vi"("error in"=w569, "data"=w571, "name"="RT: GetZeroPosOffsets", "connection info in"=w568) -> ("error out"=w566:errorcluster)  [unwired: 6 in, 1 out]
              }
              frame "PC: ViewRawPosition" {
                w580 = fxp<+/-,25,5>[] [0.0, 0.0, 0.0, 0.0, 0.0] ("PosMeas_ZeroOffset")
                n235 = To Double Precision Float(number=w580) -> (double precision float=w583:dbl[])
                n236 = xnode "Read/Write Control"("FPGA VI Reference In"=w591, "error in"=w581, "PosMeas_ZeroOffset"=w580) -> ("error out"=w585:errorcluster)  [unwired: 1 out]
                n237 = Array To Cluster(array=w583) -> (cluster=w582:T30)
                n238 = Flatten To String(anything=w582, error in (no error)=w585) -> (data string=w589:string, error out=w587:errorcluster)  [unwired: 2 in, 1 out]
                n239 = call-poly <vilib>:"Write Message.vi"("error in"=w587, "data"=w589, "name"="RT: GetZeroPosOffsets", "connection info in"=w586) -> ("error out"=w584:errorcluster)  [unwired: 6 in, 1 out]
              }
              frame "PC: ResetZeroCurrSense" {
                n240 = xnode "Read/Write Control"("FPGA VI Reference In"=w606) -> ("FPGA VI Reference Out"=w603:refnum<k20>, "error out"=w604:errorcluster, "Current Sense"=w595:fxp<+/-,25,5>[], "Current Sense Zero"=w594:fxp<+/-,25,5>[])  [unwired: 1 in]
                n241 = Add(x=w595, y=w594) -> (x+y=w593:fxp<+/-,25,5>[])
                n242 = To Double Precision Float(number=w593) -> (double precision float=w592:dbl[])
                n243 = xnode "Read/Write Control"("FPGA VI Reference In"=w603, "error in"=w604, "Current Sense Zero"=w593) -> ("error out"=w598:errorcluster)  [unwired: 1 out]
                n244 = Array To Cluster(array=w592) -> (cluster=w596:T31)
                n245 = Flatten To String(anything=w596, error in (no error)=w598) -> (data string=w602:string, error out=w600:errorcluster)  [unwired: 2 in, 1 out]
                n246 = call-poly <vilib>:"Write Message.vi"("error in"=w600, "data"=w602, "name"="RT: GetZeroCurrSense", "connection info in"=w599) -> ("error out"=w597:errorcluster)  [unwired: 6 in, 1 out]
              }
              frame "PC: UpdateReference" {
                n247 = Unflatten From String(type=T25 {"Reference Location"=enum."Pos Ref", "Direction"=enum."Z", "Excitation mode"=enum."DC", "Amplitude"=0.0, "Frequency (periods/tick)"=0.0, "PosRef_Offset"=[]} ("FuncGenParams"), binary string=w615, error in (no error)=w609) -> (value=w612:T25, error out=w610:errorcluster)  [unwired: 2 in, 1 out]
                n248 = Unbundle By Name(w612) -> ("Reference Location"=w613:T26)
                n249 = case shown="\"Pos Ref\", Default" w613 {
                  tunnel: w612 -> [w628 w647]
                  tunnel: w611 -> [w632 w651]
                  tunnel: w610 -> [w631 w650]
                  tunnel: [w630 w649] -> w608
                  frame "Ctrl Eff" {
                    n250 = Unbundle By Name(w628) -> ("Direction"=w627:T23, "Excitation mode"=w622:T27, "Amplitude"=w626:dbl, "Frequency (periods/tick)"=w625:dbl, "PosRef_Offset"=w617:dbl[])
                    n251 = for {
                      tunnel: w617 -> [w634] mode=indexing
                      tunnel: [w633] -> w618 mode=indexing
                      n252 = To Fixed-Point(number=w634) -> (fixed-point=w633:fxp<+/-,25,5>)  [unwired: 1 in]
                    }
                    n253 = To Fixed-Point(number=w626) -> (fixed-point=w621:fxp<+/-,25,5>)  [unwired: 1 in]
                    n254 = To Fixed-Point(number=w625) -> (fixed-point=w620:fxp<+,32,0>)  [unwired: 1 in]
                    n255 = Replace Array Subset(array=fxp<+/-,25,5>[] [0.0, 0.0, 0.0, 0.0, 0.0] ("Z,ThX,ThY,Bow Ref"), new element=w618) -> (w616:fxp<+/-,25,5>[])  [unwired: 1 in]
                    n256 = xnode "Read/Write Control"("FPGA VI Reference In"=w632, "error in"=w631, "Enable  Ctrl Eff dist?"=TRUE, "Select CE direction"=w627, "CE Excitation mode"=w622, "CE Amplitude [V]"=w621, "CE Frequency [periods/tick]"=w620, "Enable  Pos. Ref. Gen?"=FALSE, "Enable  AO dist?"=FALSE, "Z,ThX,ThY,B,Bd Ref"=w616) -> ("error out"=w630:errorcluster)  [unwired: 1 out]
                  }
                  frame "Pos Ref", Default {
                    n257 = Unbundle By Name(w647) -> ("Direction"=w646:T23, "Excitation mode"=w641:T27, "Amplitude"=w645:dbl, "Frequency (periods/tick)"=w644:dbl, "PosRef_Offset"=w637:dbl[])
                    n258 = for {
                      tunnel: w637 -> [w653] mode=indexing
                      tunnel: [w652] -> w636 mode=indexing
                      n259 = To Fixed-Point(number=w653) -> (fixed-point=w652:fxp<+/-,25,5>)  [unwired: 1 in]
                    }
                    n260 = To Fixed-Point(number=w645) -> (fixed-point=w640:fxp<+/-,25,5>)  [unwired: 1 in]
                    n261 = To Fixed-Point(number=w644) -> (fixed-point=w639:fxp<+,32,0>)  [unwired: 1 in]
                    n262 = Replace Array Subset(array=fxp<+/-,25,5>[] [0.0, 0.0, 0.0, 0.0, 0.0] ("Z,ThX,ThY,Bow Ref"), new element=w636) -> (w635:fxp<+/-,25,5>[])  [unwired: 1 in]
                    n263 = xnode "Read/Write Control"("FPGA VI Reference In"=w651, "error in"=w650, "Enable  Pos. Ref. Gen?"=TRUE ("Enable  Ctrl Eff dist?"), "Select Ref. direction"=w646, "PR Excitation mode"=w641, "PR Amplitude [V]"=w640, "PR Frequency [periods/tick]"=w639, "Enable  Ctrl Eff dist?"=FALSE, "Enable  AO dist?"=FALSE, "Z,ThX,ThY,B,Bd Ref"=w635) -> ("error out"=w649:errorcluster)  [unwired: 1 out]
                  }
                }
              }
              frame "PC: ShutDown" {
                # "Exit Other While Loops\nJust add an element to queue\nOther loops will execute and then \nexit since Stop variable is True!"
                n264 = shared-variable ".\\variables.lvlib\\Stop"(TRUE ("Stop"), error in=w658) -> (error out=w655:errorcluster)
                n265 = disable-structure shown="Enabled" {
                  disable-tunnel: w656 -> [w666 _]
                  disable-tunnel: w655 -> [w664 _]
                  disable-tunnel: [w663 _] -> w654
                  frame Enabled {
                    n266 = Unbundle By Name(w666) -> ("InterProcessQueue"=w667:refnum<queue>)
                    n267 = Bundle By Name(cluster=T28 {"Command"="", "Data"=variant} ("STMparseQueue"), "Command"="IP: ShutDown") -> (w668:T28)
                    n268 = Enqueue Element(queue=w667, element=w668, error in (no error)=w664) -> (error out=w663:errorcluster)  [unwired: 1 in, 2 out]
                  }
                  frame Disabled {
                  }
                }
                n269 = xnode "Read/Write Control"("FPGA VI Reference In"=w661, "Run Controller?"=FALSE, "AO enable?"=FALSE) -> ()  [unwired: 1 in, 2 out]
              }
              frame "PC: UpdateCtrlParams" {
                n270 = Unflatten From String(type=T16 {"Z-direction"={"Kp"=1.0, "Ki"=50.0, "fLPF"=0.0}, "ThX-direction"={"Kp"=1.0, "Ki"=0.0, "fLPF"=0.0}, "ThY-direction"={"Kp"=1.0, "Ki"=0.0, "fLPF"=0.0}, "Bow-direction"={"Kp"=1.0, "Ki"=0.0, "fLPF"=0.0}, "Tor-direction"={"Kp"=0.0, "Ki"=0.0, "fLPF"=0.0}} ("Controller Gains"), binary string=w678, error in (no error)=w677) -> (value=w674:T16, error out=w673:errorcluster)  [unwired: 2 in, 1 out]
                n271 = shared-variable ".\\FPGAcontrolIO.lvlib\\FPGA_CtrlLoopTime [s]"() -> (w671:dbl)  [unwired: 1 in, 1 out]
                n272 = call "UpdateCtrlParams.vi"("error in (no error)"=w673, "Ts [s]"=w671, "Controller Gains"=w674, "FPGA VI Reference In"=w670) -> ("error out"=w672:errorcluster)  [unwired: 6 in, 1 out]
              }
              frame "PC: Set RTmain_loopTime" {
                # "Set RTmain Loop Time"
                n273 = Unflatten From String(type=i64 0 ("Period"), binary string=w683, error in (no error)=w680) -> (value=w688:i64, error out=w685:errorcluster)  [unwired: 2 in, 1 out]
                n274 = Unbundle By Name(w682) -> ("InterProcessQueue"=w681:refnum<queue>)
                n275 = To Variant(anything=w688) -> (Variant=w689:variant)
                n276 = Bundle By Name(cluster=T28 {"Command"="", "Data"=variant} ("STMparseQueue"), "Command"="IP: SetTimedLoop_dt", "Data"=w689) -> (w686:T28)
                n277 = Enqueue Element(queue=w681, element=w686, error in (no error)=w685) -> (error out=w679:errorcluster)  [unwired: 1 in, 2 out]
              }
              frame "PC: StartDSA" {
                w693 = FALSE ("Enable  AO dist?")
                # "Prepare FPGA to take the DSA stimulus at \nposition reference"
                n278 = Unflatten From String(type=T19 {"DSA excitation specs"={"Initial Freq. [Hz]"=1.0, "Final Freq. [Hz]"=100.0, "# pts. in interval"=20, "Samping Time [us]"=0.0, "Amplitude"=0.0003, "Offset [V]"=0.0, "Freq Units (F: rad/s, T: Hz)"=TRUE}, "Cycle Specs"={"Cycles To \nSettle (M)"=1, "Cycles To \nCalculate (N)"=2}, "Meas. TF params"={"Direction"=enum."Z", "Tras. Func."=enum."P"}} ("DSA Config Cluster"), binary string=w703, error in (no error)=w700) -> (value=w708:T19, error out=w705:errorcluster)  [unwired: 2 in, 1 out]
                n279 = Unbundle By Name(w702) -> ("InterProcessQueue"=w701:refnum<queue>)
                n280 = To Variant(anything=w708) -> (Variant=w709:variant)
                n281 = Bundle By Name(cluster=T28 {"Command"="", "Data"=variant} ("STMparseQueue"), "Command"="IP: StartDSA", "Data"=w709) -> (w706:T28)
                n282 = Enqueue Element(queue=w701, element=w706, error in (no error)=w705) -> (error out=w697:errorcluster)  [unwired: 1 in, 2 out]
                n283 = xnode "Read/Write Control"("FPGA VI Reference In"=w698, "error in"=w697, "Enable  Pos. Ref. Gen?"=TRUE, "Select Ref. direction"=enum8{"Z", "ThX", "ThY", "Bow"}."Z", "PR Excitation mode"=enum8{"DC", "Sine", "Square", "WhiteNoise"}."DC", "Enable  AO dist?"=w693, "Enable  Ctrl Eff dist?"=w693) -> ("error out"=w692:errorcluster)  [unwired: 1 out]
              }
              frame "PC: SetFPGAPosZeroOffset" {
                # "Set PosMeas_ZeroOffset in FPGA"
                n284 = Unflatten From String(type=T29 {"V_SE"=0.0, "V_NE"=0.0, "V_NW"=0.0, "V_SW"=0.0, "V_CI"=0.0} ("Pos Zero Offsets [V]"), binary string=w718, error in (no error)=w717) -> (value=w713:T29)  [unwired: 2 in, 2 out]
                n285 = Cluster To Array(cluster=w713) -> (array=w712:dbl[])
                n286 = for {
                  tunnel: w712 -> [w721] mode=indexing
                  tunnel: [w720] -> w711 mode=indexing
                  n287 = To Fixed-Point(number=w721) -> (fixed-point=w720:fxp<+/-,25,5>)  [unwired: 1 in]
                }
                n288 = xnode "Read/Write Control"("FPGA VI Reference In"=w716, "PosMeas_ZeroOffset"=w711) -> ("error out"=w715:errorcluster)  [unwired: 1 in, 1 out]
              }
              frame "PC: StopDSA" {
                # "Clear -804 error\nif timed loop already stopped"
                # "Stop Timed Loop Structure"
                n289 = call <vilib>:"Stop Timed Structure.vi"("error in (no error)"=w726, "name"="DSAloop") -> ("error out"=w724:errorcluster)  [unwired: 9 in]
                n290 = call <vilib>:"Clear Errors.vi"("error in (no error)"=w724, "specific error code to clear (0: all)"=-804) -> ("error out"=w723:errorcluster)  [unwired: 4 in, 1 out]
              }
              frame "PC: StartPlaMoS" {
                n291 = Unflatten From String(type=T10 [] ("Planned Motion Sequence Steps"), binary string=w733, error in (no error)=w730) -> (value=w738:T10, error out=w735:errorcluster)  [unwired: 2 in, 1 out]
                n292 = Unbundle By Name(w732) -> ("InterProcessQueue"=w731:refnum<queue>)
                n293 = To Variant(anything=w738) -> (Variant=w739:variant)
                n294 = Bundle By Name(cluster=T28 {"Command"="", "Data"=variant} ("STMparseQueue"), "Command"="IP: StartPlaMoS", "Data"=w739) -> (w736:T28)
                n295 = Enqueue Element(queue=w731, element=w736, error in (no error)=w735) -> (error out=w728:errorcluster)  [unwired: 1 in, 2 out]
              }
              frame "PC: StopPlaMoS" {
                # "Clear -804 error\nif timed loop already stopped"
                # "Stop Timed Loop Structure"
                n296 = call <vilib>:"Stop Timed Structure.vi"("error in (no error)"=w745, "name"="PlaMoSloop") -> ("error out"=w743:errorcluster)  [unwired: 9 in]
                n297 = call <vilib>:"Clear Errors.vi"("error in (no error)"=w743, "specific error code to clear (0: all)"=-804) -> ("error out"=w742:errorcluster)  [unwired: 4 in, 1 out]
              }
            }
          }
          frame True {
          }
        }
      }
      frame "ShutDown" {
        n298 = call-poly <vilib>:"Write Message.vi"("error in"=w755, "name"="RT: ShutDown", "connection info in"=w756) -> ("error out"=w751:errorcluster, "connection info out"=w750:T5)  [unwired: 7 in]
        n299 = case shown="No Error" w751 {
          selector: w751 -> [w760 w763]
          tunnel: w750 -> [_ w764]
          tunnel: [w760 w762] -> w749
          frame No Error {
            # "Do nothing if no error"
          }
          frame Error {
            (unwired) T32 0 items=["no dialog", "OK message", "continue or stop message", "OK message + warnings", "continue/stop + warnings"] ("type of dialog (OK msg:1)")
            # "If error, send Error info \nto Host if possible"
            n300 = call <vilib>:"Simple Error Handler.vi"("error in (no error)"=w763) -> ("error out"=w762:errorcluster, "message"=w761:string)  [unwired: 4 in, 3 out]
            n301 = call-poly <vilib>:"Write Message.vi"("data"=w761, "name"="RT: Error", "connection info in"=w764) -> ()  [unwired: 7 in, 2 out]
          }
        }
        n302 = shared-variable ".\\variables.lvlib\\Stop"(TRUE ("Stop"), error in=w749) -> (error out=w753:errorcluster)
      }
    }
    n303 = shared-variable ".\\variables.lvlib\\Stop"() -> (w494:bool)  [unwired: 1 in, 1 out]
    n304 = Compound Arithmetic op=OR(w494, w492, w500) -> (w499:bool)
  }
  n305 = node-c288(w43) -> (w4:errorcluster)
  n306 = shared-variable ".\\variables.lvlib\\Stop"(w17) -> ()  [unwired: 1 in, 1 out]
  n307 = shared-variable ".\\variables.lvlib\\Stop"(w37) -> ()  [unwired: 1 in, 1 out]
  n308 = shared-variable ".\\variables.lvlib\\Stop"(w38) -> ()  [unwired: 1 in, 1 out]
  n309 = shared-variable ".\\variables.lvlib\\Stop"(w15) -> ()  [unwired: 1 in, 1 out]
  n310 = shared-variable ".\\variables.lvlib\\Stop"(w10) -> ()  [unwired: 1 in, 1 out]
  n311 = RT FIFO Delete(0:w35, 3:w29) -> (11:w34:errorcluster)  [unwired: 1 in]
  n312 = Merge Errors(w14, w4, w3, w2) -> (w23:errorcluster)
  n313 = xnode "Read/Write Control"("FPGA VI Reference In"=w24, "error in"=w23, "AO enable?"=FALSE, "Run Controller?"=FALSE) -> ("FPGA VI Reference Out"=w27:refnum<k20>, "error out"=w28:errorcluster)
  n314 = xnode "Close FPGA VI Reference"("FPGA VI Reference In"=w27, "error in"=w28) -> ("error out"=w7:errorcluster)
  n315 = call "Close Queues.vi"("error in (no error)"=w7, "FIFOs In"=w6) -> ("error out"=w5:errorcluster)  [unwired: 9 in]
  n316 = Merge Errors(w34, w5) -> (w22:errorcluster)
  n317 = case shown="Error .." w22 {
    selector: w22 -> [w766 w772]
    tunnel: w21 -> [w767 w775]
    tunnel: [w766 w768] -> w20
    tunnel: [w767 w774] -> w19
    frame No Error {
      # "Do nothing if no error"
    }
    frame Error {
      w773 = T32 0 items=["no dialog", "OK message", "continue or stop message", "OK message + warnings", "continue/stop + warnings"] ("type of dialog (OK msg:1)")
      # "If error, send Error info \nto Host if possible before closing"
      n318 = call <vilib>:"Simple Error Handler.vi"("type of dialog (OK msg:1)"=w773, "error in (no error)"=w772) -> ("error out"=w769:errorcluster, "message"=w771:string)  [unwired: 3 in, 3 out]
      n319 = call-poly <vilib>:"Write Message.vi"("data"=w771, "name"="RT: Error", "connection info in"=w775) -> ("error out"=w770:errorcluster, "connection info out"=w774:T5)  [unwired: 7 in]
      n320 = Merge Errors(w770, w769) -> (w768:errorcluster)
    }
  }
  n321 = call-poly <vilib>:"Get Connection Reference.vi"("error in"=w20, "connection info in"=w19) -> ("error out"=w33:errorcluster, "connection ID out"=w32:refnum<k5>)  [unwired: 7 in, 1 out]
  n322 = TCP Close Connection(connection ID=w32, error in (no error)=w33) -> (error out=w31:errorcluster)  [unwired: 1 in, 1 out]
  n323 = call "Specific Error Handler"("Error to Check"=w31) -> ("error out"=w30:errorcluster)  [unwired: 11 in, 3 out]
  n324 = call <vilib>:"Simple Error Handler.vi"("error in (no error)"=w30) -> ()  [unwired: 4 in, 5 out]
